vi "Decode MS file OCDEM.vi"() -> ()   [LabVIEW 2015]
uses:
  <vilib>/Analysis/baseanly.llb/Mean (DBL).vi
  <vilib>/Analysis/NI_AALBase.lvlib
panel:
  in  "Reference timestamp\n(i.e. time of admission for DKA)":timestamp=timestamp(3532000320 s since 1904-01-01)
  in  "Start of study":timestamp=timestamp(3532000320 s since 1904-01-01)
  out "Sum /ppb or %":dbl
  in  "Copy Button":bool
  out "Peak /ppb or %":dbl
  out "Average between cursors /ppb or %":dbl
  in  "Plot 2":u16(ring) items=["Sample1.msdat", "Sample10.msdat", "Sample11.msdat", "Sample12.msdat", "Sample2.msdat", "Sample3.msdat", "Sample4.msdat", "Sample5.msdat", "Sample6.msdat", "Sample7.msdat", "Sample8.msdat", "Sample9.msdat"]
  in  "Batch conversion":bool
  in  "Folder for batch conversion":path
  out "Concentration /ppb or %":dbl
  out "Time /s":dbl
  in  "Save":bool
  in  "Stop Button":bool
  in  "Plot":u16(ring) items=["O2 - EI", "CO2 - EI", "Ethanol", "Acetone", "Propanol", "Isoprene", "Acetol"]
  out "XY Graph":cluster{dbl[], dbl[]}(graph)
  in  "File Path Control":path
  # "Reading at red cursor"
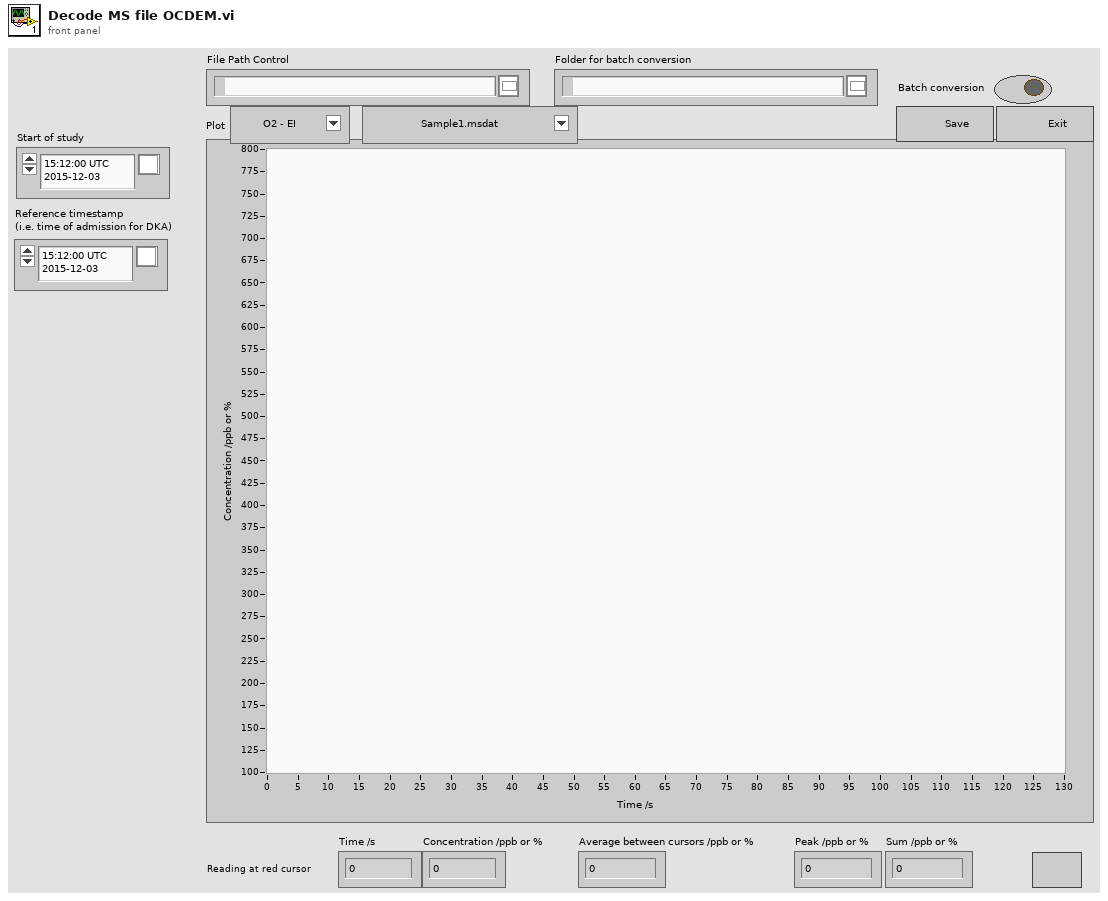
[diagram p1: front panel]
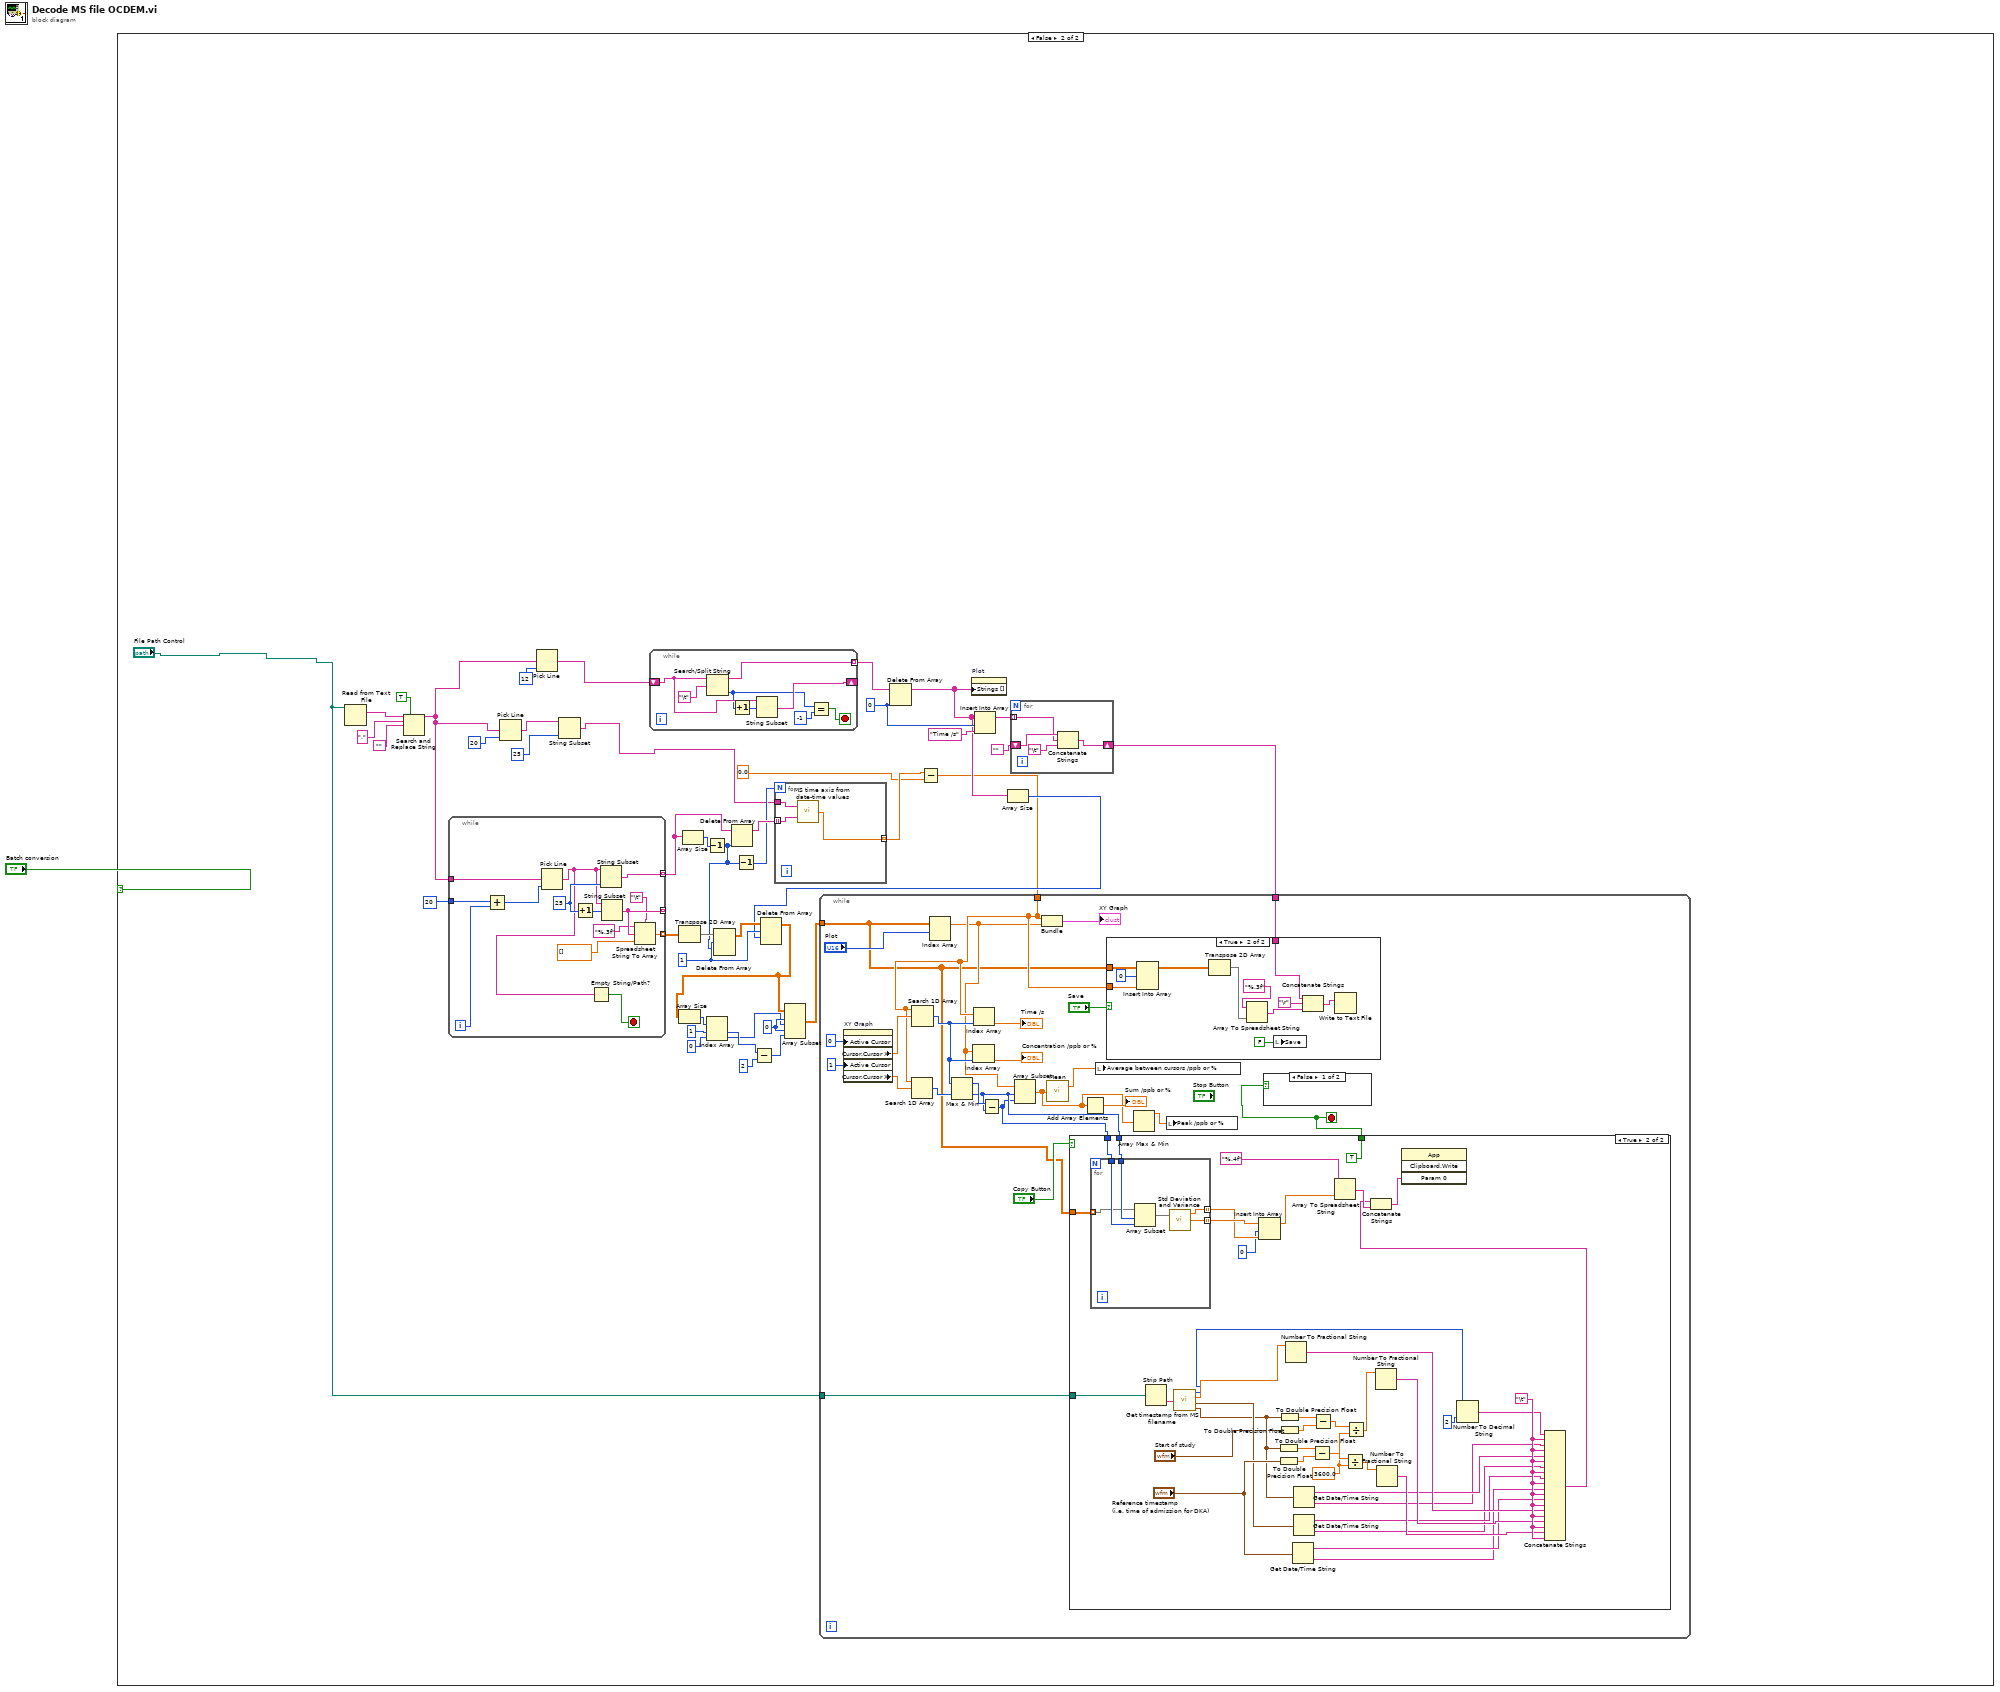
[diagram p0: block diagram]
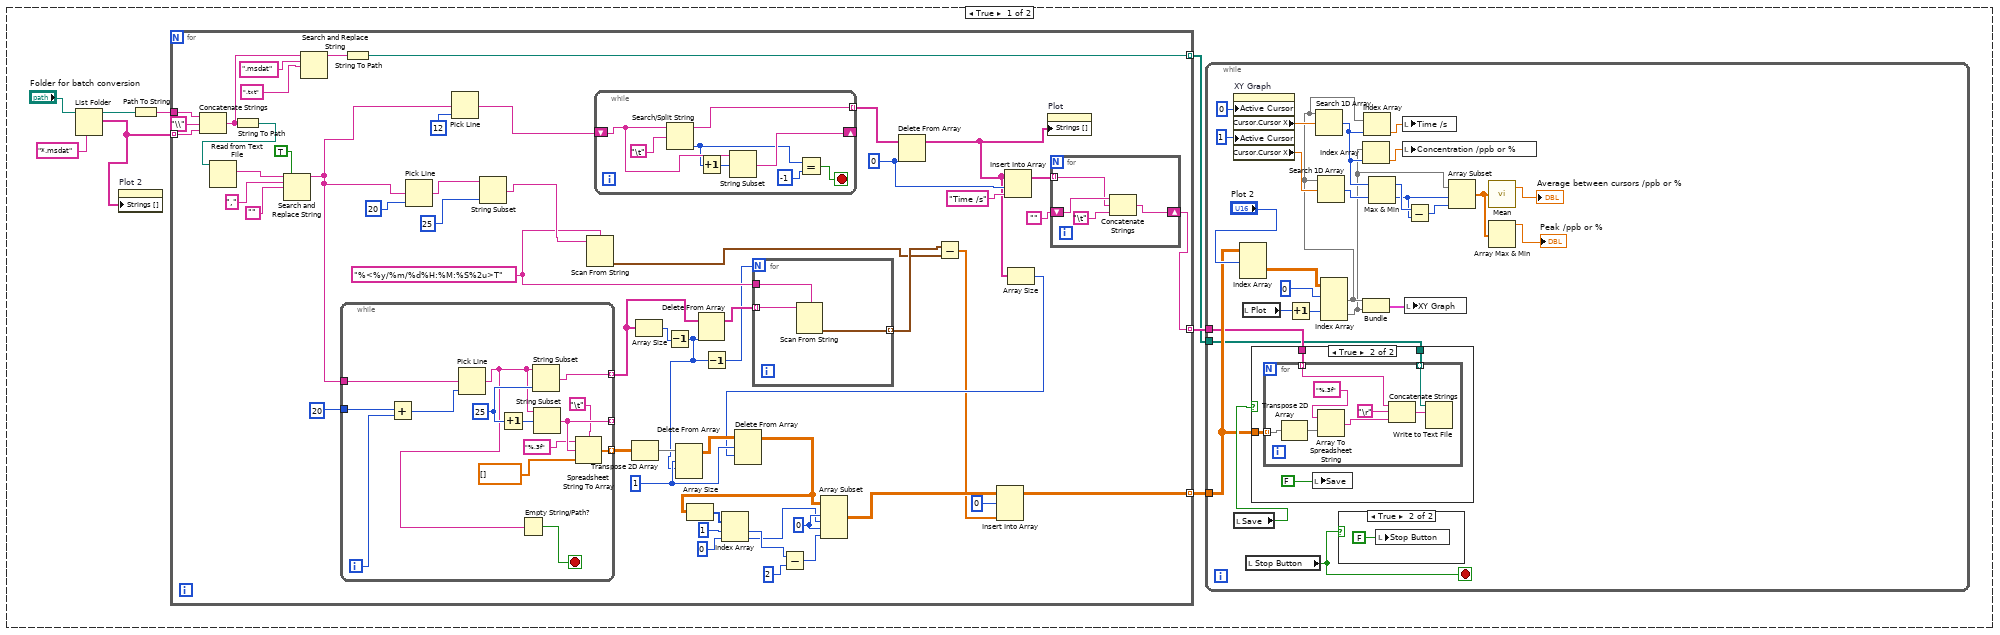
[diagram p2: hidden frame]
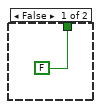
[diagram p5: hidden frame]
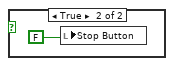
[diagram p6: hidden frame]
diagram:
  n1 = case shown="False" "Batch conversion" {
    frame True {
      n2 = List Folder(path="Folder for batch conversion", pattern="*.msdat") -> (path out=w8:path, filenames=w5:string[])  [unwired: 2 in, 2 out]
      n3 = property on="Plot 2" class="Ring (strict)"("Strings []"=w5) -> ()  [unwired: 2 in, 2 out]
      n4 = Path To String(path=w8) -> (string=w7:string)
      n5 = for {
        tunnel: w7 -> [w71]
        tunnel: w5 -> [w70] mode=indexing
        tunnel: [w52] -> w4 mode=indexing
        tunnel: [w51] -> w3 mode=indexing
        tunnel: [w50] -> w2 mode=indexing
        w57 = 0
        w82 = 1
        w88 = 0
        w97 = "%<%y/%m/%d%H:%M:%S%2u>T"
        n6 = Concatenate Strings(w71, "\\", w70) -> (w67:string)
        n7 = String To Path(string=w67) -> (path=w69:path)
        n8 = Read from Text File(file (use dialog)=w69) -> (text=w78:string)  [unwired: 3 in, 3 out]
        n9 = Search and Replace String(replace all?=TRUE, input string=w78, search string=",", replace string="") -> (result string=w75:string)  [unwired: 4 in, 3 out]
        n10 = Search and Replace String(input string=w67, search string=".msdat", replace string=".txt") -> (result string=w64:string)  [unwired: 5 in, 3 out]
        n11 = while {
          tunnel: 20 -> [w131]
          tunnel: w75 -> [w129]
          tunnel: [w124] -> w98 mode=indexing
          tunnel: [w123] -> _ mode=indexing
          tunnel: [w119] -> w93 mode=indexing
          i -> [w132]
          stop <- w128 stop-if-true
          w127 = 25
          n12 = Add(x=w131, y=w132) -> (x+y=w130:i32)
          n13 = Pick Line(multi-line string=w129, line index=w130) -> (output string=w125:string)  [unwired: 1 in]
          n14 = Increment(x=w127) -> (x+1=w126:i32)
          n15 = Empty String/Path?(string/path=w125) -> (empty?=w128:bool)
          n16 = String Subset(string=w125, length (rest)=w127) -> (substring=w124:string)  [unwired: 1 in]
          n17 = String Subset(string=w125, offset (0)=w126) -> (substring=w123:string)  [unwired: 1 in]
          n18 = Spreadsheet String To Array(delimiter (Tab)="\t", format string="%.3f", spreadsheet string=w123, array type (2D Dbl)=dbl[] []) -> (array=w119:dbl[])
        }
        n19 = String To Path(string=w64) -> (path=w50:path)
        n20 = Pick Line(multi-line string=w75, line index=20) -> (output string=w102:string)  [unwired: 1 in]
        n21 = Pick Line(multi-line string=w75, line index=12) -> (output string=w91:string)  [unwired: 1 in]
        n22 = String Subset(string=w102, length (rest)=25) -> (substring=w100:string)  [unwired: 1 in]
        n23 = Scan From String(format string=w97, input string=w100) -> (output 1=w94:timestamp)  [unwired: 3 in, 3 out]
        n24 = while {
          shift-right: [w112] -> _
          shift-left: w91 -> [w113]
          tunnel: [w114] -> w90 mode=indexing
          stop <- w111 stop-if-true
          n25 = Search/Split String(string=w113, search string/char (-)="\t") -> (substring before match=w114:string, offset of match=w109:i32)  [unwired: 1 in, 1 out]
          n26 = Increment(x=w109) -> (x+1=w108:i32)
          n27 = String Subset(string=w113, offset (0)=w108) -> (substring=w112:string)  [unwired: 1 in]
          n28 = Equal?(x=w109, y=-1) -> (x = y?=w111:bool)
        }
        n29 = Transpose 2D Array(2D array=w93) -> (transposed array=w85:dbl[][])
        n30 = Array Size(array=w98) -> (size(s)=w86:i32)
        n31 = Decrement(x=w86) -> (x-1=w80:i32)
        n32 = Delete From Array(array=w85, length=w82, index (row)=w80) -> (array with subset deleted=w84:dbl[][])  [unwired: 1 in, 1 out]
        n33 = Delete From Array(array=w98, index=w80) -> (array with subset deleted=w96:string[])  [unwired: 1 in, 1 out]
        n34 = Decrement(x=w80) -> (x-1=w79:i32)
        n35 = for {
          N: w79 -> [_]
          tunnel: w97 -> [w118]
          tunnel: w96 -> [w117] mode=indexing
          tunnel: [w116] -> w95 mode=indexing
          n36 = Scan From String(format string=w118, input string=w117) -> (output 1=w116:timestamp)  [unwired: 3 in, 3 out]
        }
        n37 = Delete From Array(array=w90, index=w88) -> (array with subset deleted=w68:string[])  [unwired: 1 in, 1 out]
        n38 = Subtract(x=w95, y=w94) -> (x-y=w55:dbl[])
        n39 = Insert Into Array(array=w68, index=w88, new element="Time /s") -> (w83:string[])
        n40 = Array Size(array=w68) -> (size(s)=w81:i32)
        n41 = Delete From Array(array=w84, length=w82, index (row)=w81) -> (array with subset deleted=w58:dbl[][])  [unwired: 1 in, 1 out]
        n42 = Array Size(array=w58) -> (size(s)=w61:i32[])
        n43 = Index Array(array=w61, index #1=1, index #2=0) -> (element #1=w60:i32, element #2=w53:i32)
        n44 = Subtract(x=w60, y=2) -> (x-y=w54:i32)
        n45 = Array Subset(array=w58, index (row)=w57, length (row)=w53, index (col)=w57, length (col)=w54) -> (w59:dbl[][])
        n46 = Insert Into Array(array=w59, index (row)=0, new element=w55) -> (w52:dbl[][])  [unwired: 1 in]
        n47 = property on="Plot" class="Ring (strict)"("Strings []"=w68) -> ()  [unwired: 2 in, 2 out]
        n48 = for {
          shift-right: [w107] -> w51
          shift-left: "" -> [w106]
          tunnel: w83 -> [w105] mode=indexing
          n49 = Concatenate Strings(w106, w105, "\t") -> (w107:string)
        }
      }
      n50 = while {
        tunnel: w4 -> [w30]
        tunnel: w3 -> [w29]
        tunnel: w2 -> [w28]
        stop <- w27 stop-if-true
        n51 = property on="XY Graph" class="XYGraph (strict)"("Active Cursor"=0, "Active Cursor"=1) -> ("Cursor.Cursor X"=w24:dbl, "Cursor.Cursor X"=w21:dbl)  [unwired: 2 in, 2 out]
        n52 = local read "Save"() -> (w31:bool)
        n53 = Index Array(array=w30, index (dim 0)="Plot 2") -> (element=w12:dbl[][])  [unwired: 2 in]
        n54 = local read "Plot"() -> (w34:u16)
        n55 = local read "Stop Button"() -> (w27:bool)
        n56 = case shown="True" w31 {
          tunnel: w30 -> [_ w41]
          tunnel: w29 -> [_ w40]
          tunnel: w28 -> [_ w39]
          frame False {
          }
          frame True {
            n57 = for {
              tunnel: w41 -> [w44] mode=indexing
              tunnel: w40 -> [w43] mode=indexing
              tunnel: w39 -> [w42] mode=indexing
              n58 = Transpose 2D Array(2D array=w44) -> (transposed array=w45:dbl[][])
              n59 = Array To Spreadsheet String(array=w45, 3:"%.3f") -> (spreadsheet string=w48:string)  [unwired: 1 in]
              n60 = Concatenate Strings(w43, "\r", w48) -> (w46:string)
              n61 = Write to Text File(file (use dialog)=w42, text=w46) -> ()  [unwired: 2 in, 3 out]
            }
            n62 = local write "Save"(FALSE) -> ()
          }
        }
        n63 = Increment(x=w34) -> (x+1=w35:u16)
        n64 = Index Array(array=w12, index (row) #1=0, index (row) #2=w35) -> (element #1=w20:dbl[], element #2=w16:dbl[])  [unwired: 2 in]
        n65 = Search 1D Array(1D array=w20, element=w24) -> (index of element=w18:i32)  [unwired: 1 in]
        n66 = Search 1D Array(1D array=w20, element=w21) -> (index of element=w19:i32)  [unwired: 1 in]
        n67 = case shown="True" w27 {
          frame False {
          }
          frame True {
            n68 = local write "Stop Button"(FALSE) -> ()
          }
        }
        n69 = Index Array(array=w16, index=w18) -> (element=w22:dbl)
        n70 = Bundle(w20, w16) -> (w36:cluster{dbl[], dbl[]})  [unwired: 1 in]
        n71 = Index Array(array=w20, index=w18) -> (element=w23:dbl)
        n72 = Max & Min(x=w18, y=w19) -> (max(x,y)=w17:i32, min(x,y)=w11:i32)
        n73 = local write "Time /s"(w23) -> ()
        n74 = local write "Concentration /ppb or %"(w22) -> ()
        n75 = local write "XY Graph"(w36) -> ()
        n76 = Subtract(x=w17, y=w11) -> (x-y=w10:i32)
        n77 = Array Subset(array=w16, index=w11, length=w10) -> (w14:dbl[])
        n78 = call-poly <vilib>:"Mean.vi"("X"=w14) -> ("mean"=→"Average between cursors /ppb or %":dbl)  [unwired: 1 out]
        n79 = Array Max & Min(array=w14) -> (max value=→"Peak /ppb or %":dbl)  [unwired: 3 out]
      }
    }
    frame False {
      w142 = 0
      w155 = 1
      w163 = 0
      n80 = Read from Text File(file (use dialog)="File Path Control") -> (text=w136:string)  [unwired: 3 in, 3 out]
      n81 = Search and Replace String(replace all?=TRUE, input string=w136, search string=",", replace string="") -> (result string=w149:string)  [unwired: 4 in, 3 out]
      n82 = while {
        tunnel: 20 -> [w288]
        tunnel: w149 -> [w286]
        tunnel: [w281] -> w171 mode=indexing
        tunnel: [w280] -> _ mode=indexing
        tunnel: [w276] -> w168 mode=indexing
        i -> [w289]
        stop <- w285 stop-if-true
        w284 = 25
        n83 = Add(x=w288, y=w289) -> (x+y=w287:i32)
        n84 = Pick Line(multi-line string=w286, line index=w287) -> (output string=w282:string)  [unwired: 1 in]
        n85 = Increment(x=w284) -> (x+1=w283:i32)
        n86 = Empty String/Path?(string/path=w282) -> (empty?=w285:bool)
        n87 = String Subset(string=w282, length (rest)=w284) -> (substring=w281:string)  [unwired: 1 in]
        n88 = String Subset(string=w282, offset (0)=w283) -> (substring=w280:string)  [unwired: 1 in]
        n89 = Spreadsheet String To Array(delimiter (Tab)="\t", format string="%.3f", spreadsheet string=w280, array type (2D Dbl)=dbl[] []) -> (array=w276:dbl[])
      }
      n90 = Pick Line(multi-line string=w149, line index=20) -> (output string=w174:string)  [unwired: 1 in]
      n91 = Pick Line(multi-line string=w149, line index=12) -> (output string=w166:string)  [unwired: 1 in]
      n92 = String Subset(string=w174, length (rest)=25) -> (substring=w133:string)  [unwired: 1 in]
      n93 = while {
        shift-right: [w269] -> _
        shift-left: w166 -> [w270]
        tunnel: [w271] -> w165 mode=indexing
        stop <- w268 stop-if-true
        n94 = Search/Split String(string=w270, search string/char (-)="\t") -> (substring before match=w271:string, offset of match=w266:i32)  [unwired: 1 in, 1 out]
        n95 = Increment(x=w266) -> (x+1=w265:i32)
        n96 = String Subset(string=w270, offset (0)=w265) -> (substring=w269:string)  [unwired: 1 in]
        n97 = Equal?(x=w266, y=-1) -> (x = y?=w268:bool)
      }
      n98 = Transpose 2D Array(2D array=w168) -> (transposed array=w159:dbl[][])
      n99 = Array Size(array=w171) -> (size(s)=w160:i32)
      n100 = Decrement(x=w160) -> (x-1=w153:i32)
      n101 = Delete From Array(array=w159, length=w155, index (row)=w153) -> (array with subset deleted=w158:dbl[][])  [unwired: 1 in, 1 out]
      n102 = Delete From Array(array=w171, index=w153) -> (array with subset deleted=w170:string[])  [unwired: 1 in, 1 out]
      n103 = Decrement(x=w153) -> (x-1=w152:i32)
      n104 = for {
        N: w152 -> [_]
        tunnel: w133 -> [w275]
        tunnel: w170 -> [w274] mode=indexing
        tunnel: [w273] -> w169 mode=indexing
        n105 = call "MS time axis from date-time values.vi"("Reference"=w275, "Time"=w274) -> ("dt /s"=w273:dbl)  [unwired: 2 out]
      }
      n106 = Delete From Array(array=w165, index=w163) -> (array with subset deleted=w156:string[])  [unwired: 1 in, 1 out]
      n107 = Subtract(x=w169, y=0.0) -> (x-y=w147:dbl[])
      n108 = property on="Plot" class="Ring (strict)"("Strings []"=w156) -> ()  [unwired: 2 in, 2 out]
      n109 = Insert Into Array(array=w156, index=w163, new element="Time /s") -> (w157:string[])
      n110 = Array Size(array=w156) -> (size(s)=w154:i32)
      n111 = Delete From Array(array=w158, length=w155, index (row)=w154) -> (array with subset deleted=w137:dbl[][])  [unwired: 1 in, 1 out]
      n112 = Array Size(array=w137) -> (size(s)=w144:i32[])
      n113 = Index Array(array=w144, index #1=1, index #2=0) -> (element #1=w143:i32, element #2=w139:i32)
      n114 = Subtract(x=w143, y=2) -> (x-y=w140:i32)
      n115 = Array Subset(array=w137, index (row)=w142, length (row)=w139, index (col)=w142, length (col)=w140) -> (w138:dbl[][])
      n116 = for {
        shift-right: [w179] -> w161
        shift-left: "" -> [w178]
        tunnel: w157 -> [w177] mode=indexing
        n117 = Concatenate Strings(w178, w177, "\t") -> (w179:string)
      }
      n118 = while {
        tunnel: w147 -> [w193]
        tunnel: w138 -> [w187]
        tunnel: w161 -> [w200]
        tunnel: "File Path Control" -> [w180]
        stop <- w181 stop-if-true
        n119 = property on="XY Graph" class="XYGraph (strict)"("Active Cursor"=0, "Active Cursor"=1) -> ("Cursor.Cursor X"=w198:dbl, "Cursor.Cursor X"=w194:dbl)  [unwired: 2 in, 2 out]
        n120 = Search 1D Array(1D array=w193, element=w194) -> (index of element=w196:i32)  [unwired: 1 in]
        n121 = Search 1D Array(1D array=w193, element=w198) -> (index of element=w192:i32)  [unwired: 1 in]
        n122 = Index Array(array=w187, index (row)="Plot") -> (element=w190:dbl[])  [unwired: 1 in]
        n123 = Max & Min(x=w192, y=w196) -> (max(x,y)=w191:i32, min(x,y)=w186:i32)
        n124 = Index Array(array=w190, index=w192) -> (element=→"Concentration /ppb or %":dbl)
        n125 = Index Array(array=w193, index=w192) -> (element=→"Time /s":dbl)
        n126 = Subtract(x=w191, y=w186) -> (x-y=w185:i32)
        n127 = Array Subset(array=w190, index=w186, length=w185) -> (w182:dbl[])
        n128 = Bundle(w193, w190) -> (→"XY Graph":cluster{dbl[], dbl[]})  [unwired: 1 in]
        n129 = call-poly <vilib>:"Mean.vi"("X"=w182) -> ("mean"=w189:dbl)  [unwired: 1 out]
        n130 = case shown="True" "Copy Button" {
          tunnel: w186 -> [_ w246]
          tunnel: w185 -> [_ w245]
          tunnel: w187 -> [_ w244]
          tunnel: [FALSE TRUE] -> w181
          tunnel: w180 -> [_ w207]
          frame False {
          }
          frame True {
            w218 = 3600.0
            w235 = "\t"
            n131 = for {
              tunnel: w244 -> [w250] mode=indexing
              tunnel: w246 -> [w252]
              tunnel: w245 -> [w251]
              tunnel: [w248] -> w239 mode=indexing
              tunnel: [w247] -> w240 mode=indexing
              n132 = Array Subset(array=w250, index=w252, length=w251) -> (w249:dbl[])
              n133 = call <vilib>:"Std Deviation and Variance.vi"("X"=w249) -> ("mean"=w248:dbl, "standard deviation"=w247:dbl)  [unwired: 1 in, 1 out]
            }
            n134 = Strip Path(path=w207) -> (name=w208:string)  [unwired: 1 out]
            n135 = call "Get timestamp from MS filename.vi"("Filename"=w208) -> ("Subject"=w220:i32, "Sample age /hours"=w229:dbl, "Measurement Time Stamp"=w215:timestamp, "Sample Time Stamp"=w214:timestamp)
            n136 = Insert Into Array(array=w240, index=0, new element=w239) -> (w237:dbl[])
            n137 = To Double Precision Float(number=w214) -> (double precision float=w211:dbl)
            n138 = To Double Precision Float(number="Reference timestamp\n(i.e. time of admission for DKA)") -> (double precision float=w213:dbl)
            n139 = To Double Precision Float(number=w214) -> (double precision float=w210:dbl)
            n140 = To Double Precision Float(number="Start of study") -> (double precision float=w212:dbl)
            n141 = Number To Fractional String(number=w229) -> (F-format string=w230:string)  [unwired: 3 in]
            n142 = Get Date/Time String(seconds (now)="Reference timestamp\n(i.e. time of admission for DKA)") -> (date string=w228:string, time string=w227:string)  [unwired: 2 in]
            n143 = Get Date/Time String(seconds (now)=w214) -> (date string=w224:string, time string=w223:string)  [unwired: 2 in]
            n144 = Get Date/Time String(seconds (now)=w215) -> (date string=w226:string, time string=w225:string)  [unwired: 2 in]
            n145 = Subtract(x=w211, y=w213) -> (x-y=w219:dbl)
            n146 = Subtract(x=w210, y=w212) -> (x-y=w217:dbl)
            n147 = Array To Spreadsheet String(array=w237, 3:"%.4f") -> (spreadsheet string=w242:string)  [unwired: 1 in]
            n148 = Divide(x=w219, y=w218) -> (x/y=w232:dbl)
            n149 = Divide(x=w217, y=w218) -> (x/y=w231:dbl)
            n150 = Number To Fractional String(number=w231) -> (F-format string=w233:string)  [unwired: 3 in]
            n151 = Number To Fractional String(number=w232) -> (F-format string=w234:string)  [unwired: 3 in]
            n152 = Number To Decimal String(number=w220, width (-)=2) -> (decimal integer string=w222:string)
            n153 = Concatenate Strings(w222, w235, w223, w235, w224, w235, w225, w235, w226, w235, w227, w235, w228, w235, w230, w235, w233, w235, w234, w235) -> (w206:string)
            n154 = Concatenate Strings(w206, w242) -> (w241:string)
            n155 = invoke class="App" method="Clipboard.Write"("Param 0"=w241) -> ()  [unwired: 3 in, 4 out]
          }
        }
        n156 = Add Array Elements(numeric array=w182) -> (sum=→"Sum /ppb or %":dbl)
        n157 = local write "Average between cursors /ppb or %"(w189) -> ()
        n158 = case shown="True" "Save" {
          tunnel: w187 -> [_ w264]
          tunnel: w193 -> [_ w256]
          tunnel: w200 -> [_ w258]
          frame False {
          }
          frame True {
            n159 = Insert Into Array(array=w264, index (row)=0, new element=w256) -> (w255:dbl[][])  [unwired: 1 in]
            n160 = Transpose 2D Array(2D array=w255) -> (transposed array=w262:dbl[][])
            n161 = Array To Spreadsheet String(array=w262, 3:"%.3f") -> (spreadsheet string=w260:string)  [unwired: 1 in]
            n162 = local write "Save"(FALSE) -> ()
            n163 = Concatenate Strings(w258, "\r", w260) -> (w257:string)
            n164 = Write to Text File(text=w257) -> ()  [unwired: 3 in, 3 out]
          }
        }
        n165 = Array Max & Min(array=w182) -> (max value=w183:dbl)  [unwired: 3 out]
        n166 = local write "Peak /ppb or %"(w183) -> ()
        n167 = case shown="False" w181 {
          frame False {
          }
          frame True {
            n168 = local write "Stop Button"(FALSE) -> ()
          }
        }
      }
    }
  }
